vi "generateBarPosAreaQuad.vi"(7 "Number of Defenders\nWithout Duelist":i32, 8 "error in (no error)":errorcluster, 10 "Game":refnum<class "Game.lvclass">, 11 "Utilities in":refnum<class "Utilities.lvclass">) -> (0 "error out":errorcluster, 1 "Pos Centers Back":dbl[][](array[numeric]), 2 "Game out":refnum<class "Game.lvclass">, 3 "Utilities out":refnum<class "Utilities.lvclass">)   [LabVIEW 2020, in "Utilities.lvclass"]
uses:
  Utilities.lvclass
  Game_class/Game.lvclass
  Game_class/Game.lvclass/Game.ctl
  Events_class/Events.lvclass/Events.ctl
  Object_class/Object.lvclass/Object.ctl
  Game_class/Read EventsRef.vi
  Game_class/Read FieldRef.vi
  Game_class/Read BallRef.vi
  Object_class/Read x.vi
  Object_class/Read y.vi
  Events_class/Read ball_out.vi
  Events_class/Read ball_out_of_vision.vi
  Ball_class/Ball.lvclass
  Events_class/Events.lvclass
  Field_class/Field.lvclass
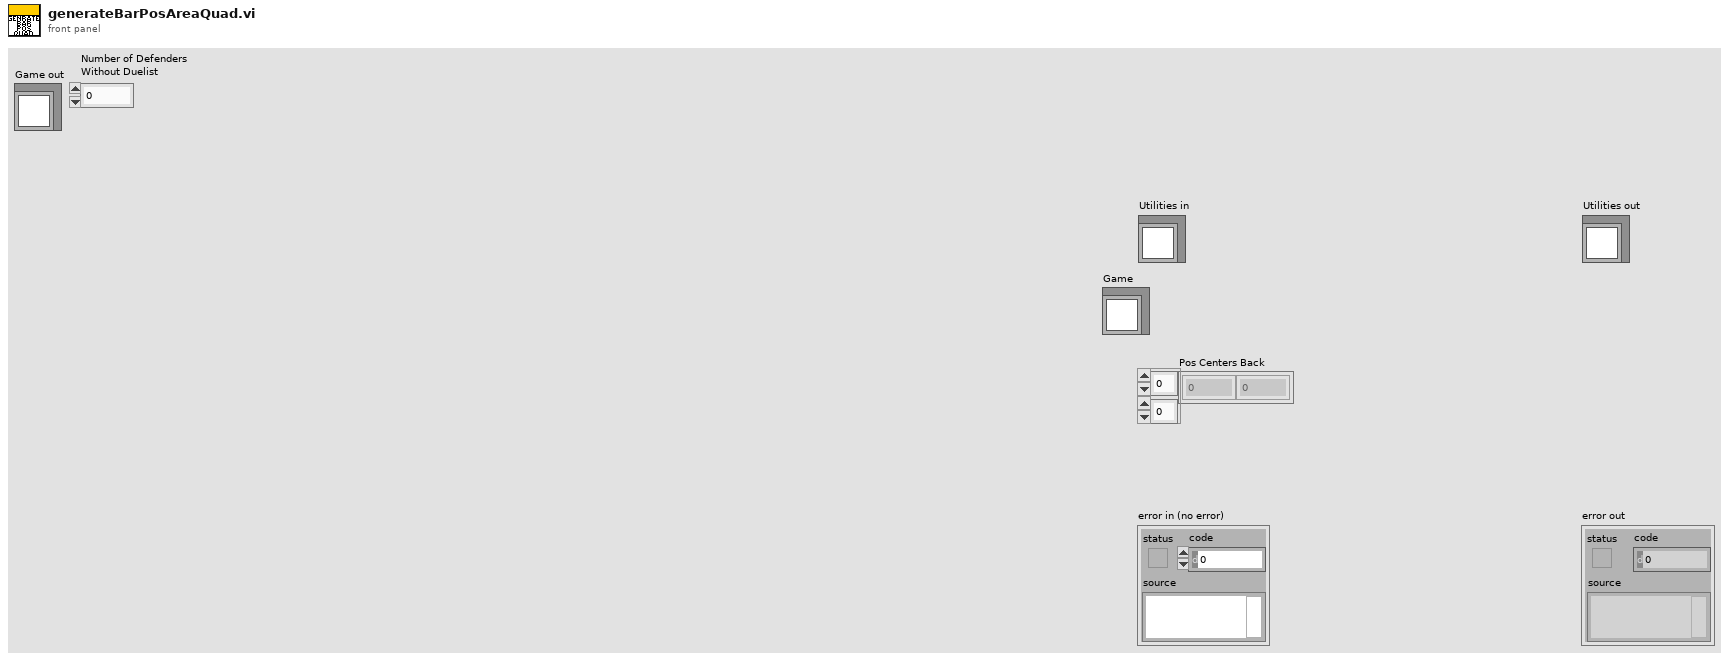
[diagram p1: front panel]
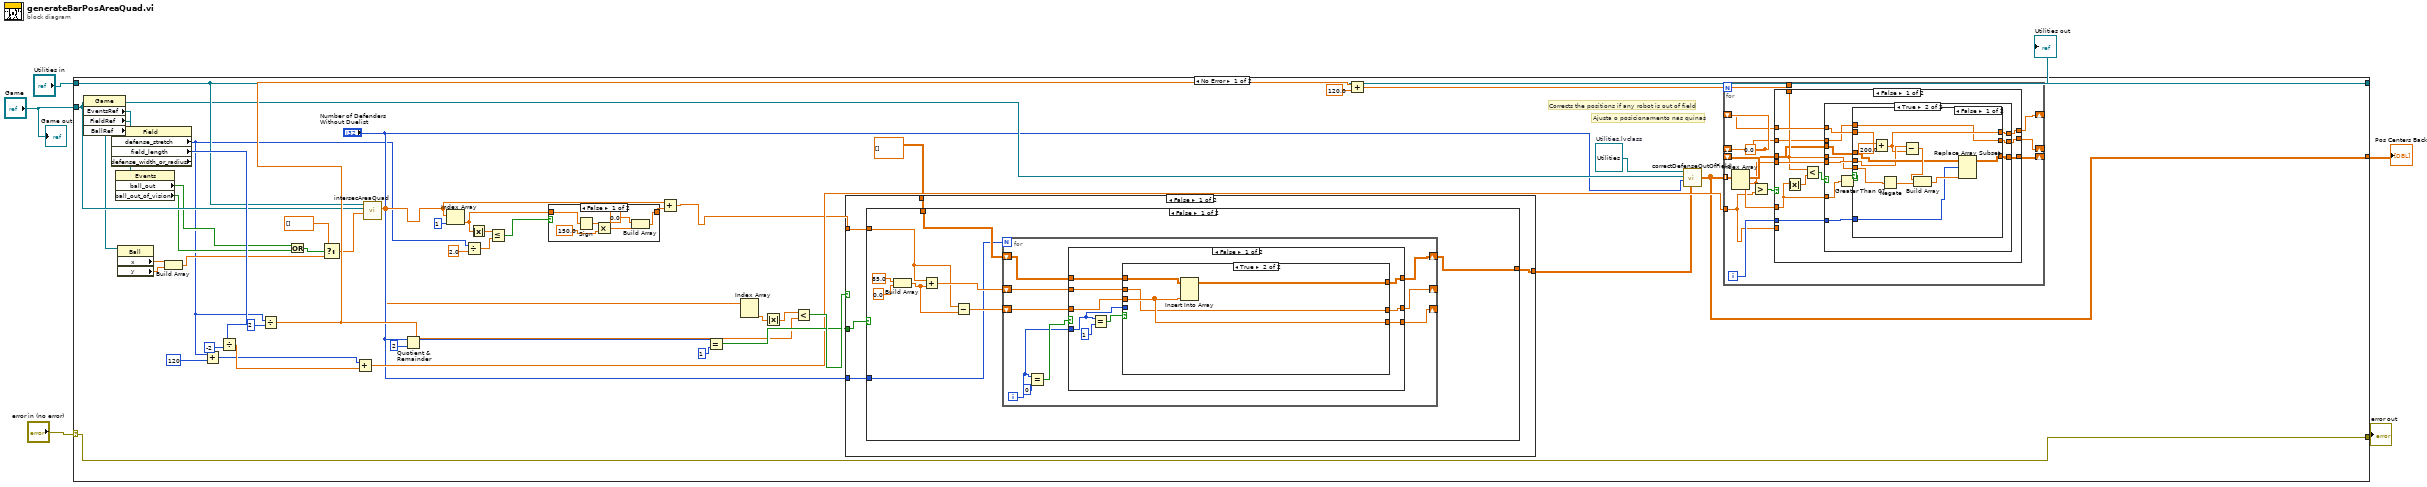
[diagram p0: block diagram]
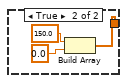
[diagram p2: hidden frame]
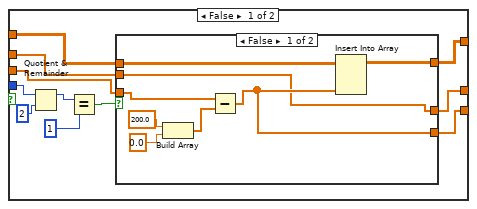
[diagram p3: hidden frame]
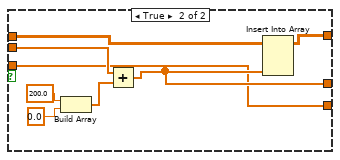
[diagram p4: hidden frame]
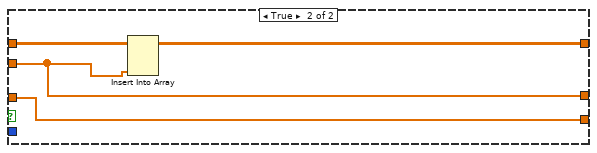
[diagram p5: hidden frame]
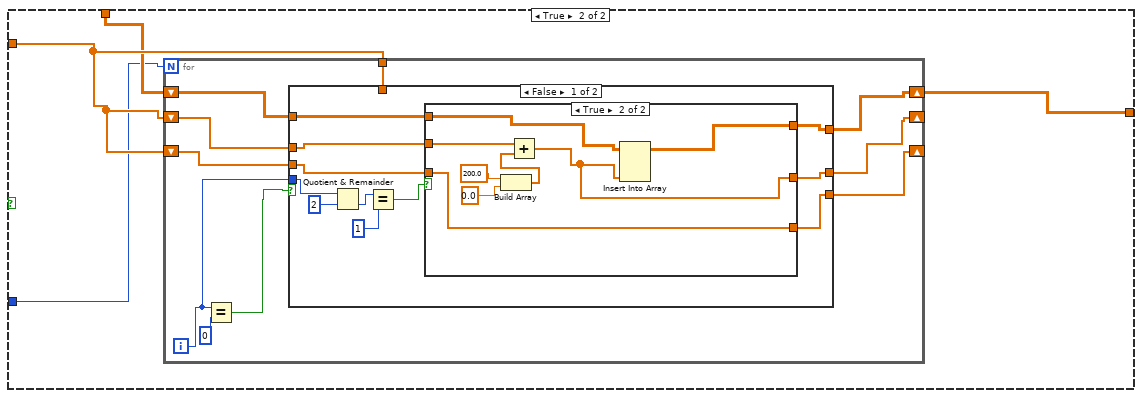
[diagram p6: hidden frame]
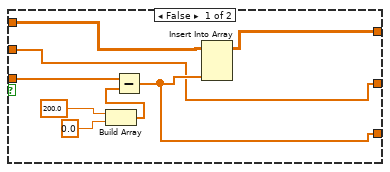
[diagram p7: hidden frame]
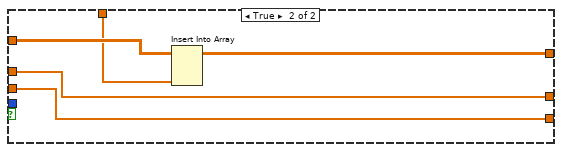
[diagram p8: hidden frame]
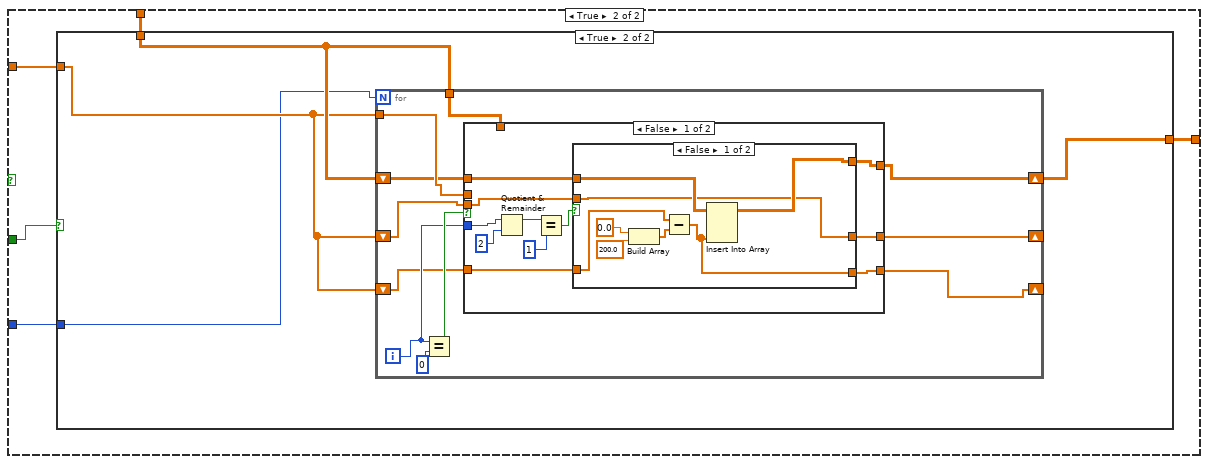
[diagram p9: hidden frame]
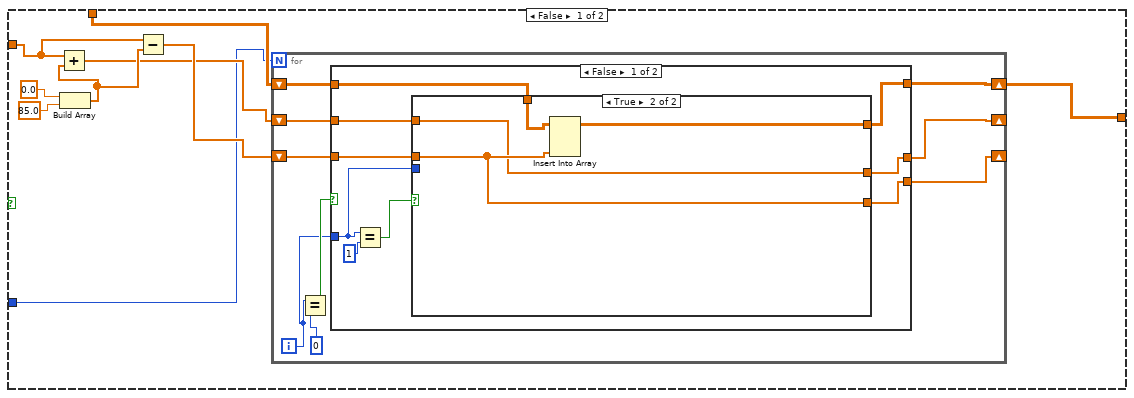
[diagram p10: hidden frame]
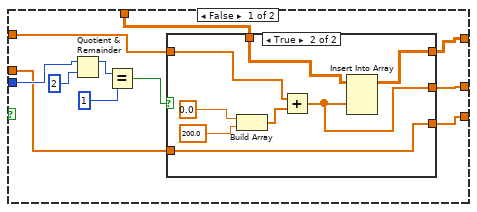
[diagram p11: hidden frame]
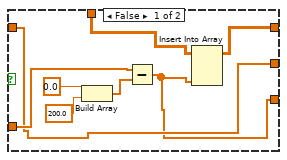
[diagram p12: hidden frame]
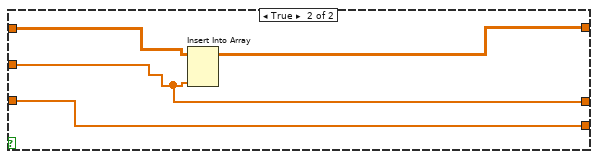
[diagram p13: hidden frame]
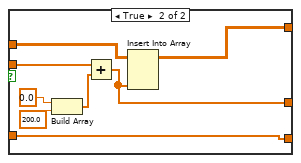
[diagram p14: hidden frame]
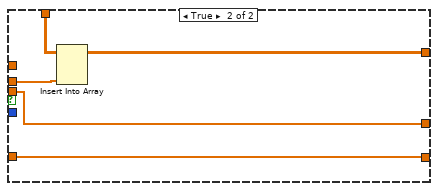
[diagram p15: hidden frame]
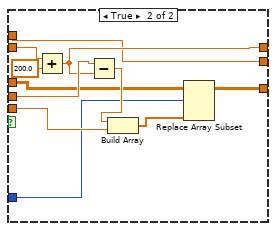
[diagram p17: hidden frame]
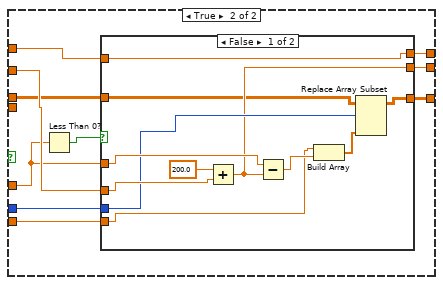
[diagram p18: hidden frame]
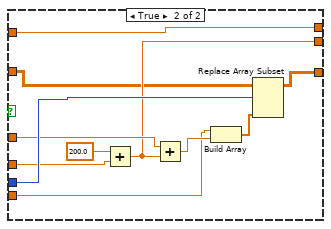
[diagram p19: hidden frame]
diagram:
  n1 = case shown="No Error" "error in (no error)" {
    selector: "error in (no error)" -> [w53 w385]
    tunnel: [w53 w385] -> w5
    tunnel: "Utilities in" -> [w33 w384]
    tunnel: [w33 w384] -> w3
    tunnel: "Game" -> [w29 _]
    tunnel: [w7 _] -> w2
    frame No Error {
      w30 = refnum<class "Utilities.lvclass"> refnum  # Utilities.lvclass
      w43 = 0.0
      # "Ajusta o posicionamento nas quinas"
      # "Corrects the positions if any robot is out of field"
      n2 = property class="Game"(reference=w29) -> ("EventsRef"=w25:refnum<class "Events.lvclass">, "FieldRef"=w35:refnum<class "Field.lvclass">, "BallRef"=w28:refnum<class "Ball.lvclass">)  [unwired: 1 in, 2 out]
      n3 = property class="Field" props=["defense_stretch", "field_length", "defense_width_or_radius"](reference=w35) -> ("defense_stretch"=w8:i32, "field_length"=w34:i32)  [unwired: 1 in, 3 out]
      n4 = property class="Events"(reference=w25) -> ("ball_out"=w24:bool, "ball_out_of_vision"=w23:bool)  [unwired: 1 in, 2 out]
      n5 = property class="Ball"(reference=w28) -> ("x"=w27:dbl, "y"=w26:dbl)  [unwired: 1 in, 2 out]
      n6 = Build Array(w27, w26) -> (w21:dbl[])
      n7 = Add(x=w8, y=u32 120) -> (x+y=w37:u32)
      n8 = Divide(x=w34, y=-2) -> (x/y=w40:dbl)
      n9 = Divide(x=w8, y=u32 2) -> (x/y=w38:dbl)
      n10 = Or(x=w24, y=w23) -> (x .or. y?=w22:bool)
      n11 = Select(t=dbl[] [], s=w22, f=w21) -> (s? t:f=w20:dbl[])
      n12 = Add(x=w37, y=w40) -> (x+y=w41:dbl)
      n13 = call "intersecAreaQuad.vi"("Ball/Enemy\nPosition"=w20, "Game"=w29, "Utilities in"=w33) -> ("Pos de Interseção"=w10:dbl[])  [unwired: 6 in, 2 out]
      n14 = Quotient & Remainder(x="Number of Defenders\nWithout Duelist", y=2) -> (x-y*floor(x/y)=w47:i32)  [unwired: 1 out]
      n15 = Index Array(array=w10, index=1) -> (element=w11:dbl)
      n16 = Divide(x=w8, y=2.0) -> (x/y=w14:dbl)
      n17 = Absolute Value(x=w11) -> (abs(x)=w15:dbl)
      n18 = Less Or Equal?(x=w15, y=w14) -> (x <= y?=w12:bool)
      n19 = case shown="False" w12 {
        tunnel: [w58 w62] -> w17
        tunnel: w11 -> [w54 _]
        frame False {
          n20 = Sign(1:w54) -> (0:w57:dbl)
          n21 = Multiply(x=w57, y=150.0) -> (x*y=w55:dbl)
          n22 = Build Array(0.0, w55) -> (w58:dbl[])
        }
        frame True {
          n23 = Build Array(150.0, 0.0) -> (w62:dbl[])
        }
      }
      n24 = Add(x=w10, y=w17) -> (x+y=w9:dbl[])
      n25 = Equal?(x=w47, y=1) -> (x = y?=w45:bool)
      n26 = Index Array(array=w10) -> (element #2=w51:dbl)  [unwired: 2 in, 1 out]
      n27 = Absolute Value(x=w51) -> (abs(x)=w50:dbl)
      n28 = Less?(x=w50, y=w38) -> (x < y?=w49:bool)
      n29 = case shown="False" w49 {
        tunnel: w45 -> [w67 w180]
        tunnel: w9 -> [w66 w179]
        tunnel: dbl[][] [] -> [w64 w178]
        tunnel: [w65 w177] -> w31
        tunnel: "Number of Defenders\nWithout Duelist" -> [w63 w176]
        frame False {
          n30 = case shown="False" w67 {
            tunnel: w64 -> [w70 w131]
            tunnel: w66 -> [w73 w133]
            tunnel: [w69 w132] -> w65
            tunnel: w63 -> [w68 w130]
            frame False {
              n31 = Build Array(85.0, 0.0) -> (w72:dbl[])
              n32 = Add(x=w73, y=w72) -> (x+y=w74:dbl[])
              n33 = Subtract(x=w73, y=w72) -> (x-y=w71:dbl[])
              n34 = for {
                N: w68 -> [_]
                shift-right: [w80] -> _
                shift-left: w74 -> [w82]
                shift-right: [w79] -> _
                shift-left: w71 -> [w78]
                shift-right: [w81] -> w69
                shift-left: w70 -> [w83]
                i -> [w77]
                n35 = Equal?(x=w77, y=0) -> (x = y?=w84:bool)
                n36 = case shown="False" w84 {
                  tunnel: w83 -> [w92 w129]
                  tunnel: w82 -> [w88 w127]
                  tunnel: [w87 w128] -> w81
                  tunnel: [w89 w127] -> w80
                  tunnel: [w90 w126] -> w79
                  tunnel: w78 -> [w91 w126]
                  tunnel: w77 -> [w86 _]
                  frame False {
                    n37 = Equal?(x=w86, y=1) -> (x = y?=w93:bool)
                    n38 = case shown="True" w93 {
                      tunnel: w92 -> [w100 w125]
                      tunnel: w91 -> [w95 w124]
                      tunnel: [w96 w124] -> w90
                      tunnel: [w97 w123] -> w89
                      tunnel: w88 -> [w99 w123]
                      tunnel: [w98 w122] -> w87
                      tunnel: w86 -> [w105 _]
                      frame False {
                        n39 = Quotient & Remainder(x=w105, y=2) -> (x-y*floor(x/y)=w103:i32)  [unwired: 1 out]
                        n40 = Equal?(x=w103, y=1) -> (x = y?=w101:bool)
                        n41 = case shown="False" w101 {
                          tunnel: w100 -> [w112 w121]
                          tunnel: w99 -> [w106 w117]
                          tunnel: [w113 w116] -> w98
                          tunnel: [w106 w115] -> w97
                          tunnel: [w107 w114] -> w96
                          tunnel: w95 -> [w108 w114]
                          frame False {
                            n42 = Build Array(200.0, 0.0) -> (w109:dbl[])
                            n43 = Subtract(x=w108, y=w109) -> (x-y=w107:dbl[])
                            n44 = Insert Into Array(array=w112, new element=w107) -> (w113:dbl[][])  [unwired: 2 in]
                          }
                          frame True {
                            n45 = Build Array(200.0, 0.0) -> (w118:dbl[])
                            n46 = Add(x=w117, y=w118) -> (x+y=w115:dbl[])
                            n47 = Insert Into Array(array=w121, new element=w115) -> (w116:dbl[][])  [unwired: 2 in]
                          }
                        }
                      }
                      frame True {
                        n48 = Insert Into Array(array=w125, new element=w124) -> (w122:dbl[][])  [unwired: 2 in]
                      }
                    }
                  }
                  frame True {
                    n49 = Insert Into Array(array=w129, new element=w127) -> (w128:dbl[][])  [unwired: 2 in]
                  }
                }
              }
            }
            frame True {
              n50 = for {
                N: w130 -> [_]
                shift-right: [w139] -> w132
                shift-left: w131 -> [w141]
                shift-right: [w137] -> _
                shift-left: w133 -> [w136]
                shift-right: [w135] -> _
                shift-left: w133 -> [w134]
                tunnel: w133 -> [w140]
                i -> [w138]
                n51 = Equal?(x=w138, y=0) -> (x = y?=w142:bool)
                n52 = case shown="False" w142 {
                  tunnel: w141 -> [w149 w175]
                  tunnel: w140 -> [_ w174]
                  tunnel: [w148 w173] -> w139
                  tunnel: w138 -> [w154 _]
                  tunnel: [w145 w172] -> w137
                  tunnel: w136 -> [w150 w172]
                  tunnel: [w146 w171] -> w135
                  tunnel: w134 -> [w147 w171]
                  frame False {
                    n53 = Quotient & Remainder(x=w154, y=2) -> (floor(x/y)=w152:i32)  [unwired: 1 out]
                    n54 = Equal?(x=w152, y=1) -> (x = y?=w144:bool)
                    n55 = case shown="True" w144 {
                      tunnel: w150 -> [w156 w168]
                      tunnel: w149 -> [w159 w166]
                      tunnel: [w158 w165] -> w148
                      tunnel: w147 -> [w160 w164]
                      tunnel: [w157 w164] -> w146
                      tunnel: [w156 w163] -> w145
                      frame False {
                        n56 = Build Array(200.0, 0.0 ("element")) -> (w161:dbl[])
                        n57 = Subtract(x=w160, y=w161) -> (x-y=w157:dbl[])
                        n58 = Insert Into Array(array=w159, new element=w157) -> (w158:dbl[][])  [unwired: 2 in]
                      }
                      frame True {
                        n59 = Build Array(200.0, 0.0) -> (w167:dbl[])
                        n60 = Add(x=w168, y=w167) -> (x+y=w163:dbl[])
                        n61 = Insert Into Array(array=w166, new element=w163) -> (w165:dbl[][])  [unwired: 2 in]
                      }
                    }
                  }
                  frame True {
                    n62 = Insert Into Array(array=w175, new element=w174) -> (w173:dbl[][])  [unwired: 2 in]
                  }
                }
              }
            }
          }
        }
        frame True {
          n63 = case shown="True" w180 {
            tunnel: w179 -> [w187 w245]
            tunnel: w178 -> [w182 w246]
            tunnel: [w183 w244] -> w177
            tunnel: w176 -> [w181 w243]
            frame False {
              n64 = Build Array(0.0, 85.0) -> (w186:dbl[])
              n65 = Add(x=w187, y=w186) -> (x+y=w184:dbl[])
              n66 = Subtract(x=w187, y=w186) -> (x-y=w185:dbl[])
              n67 = for {
                N: w181 -> [_]
                shift-right: [w190] -> _
                shift-left: w184 -> [w195]
                shift-right: [w194] -> w183
                shift-left: w182 -> [w196]
                shift-right: [w191] -> _
                shift-left: w185 -> [w192]
                i -> [w193]
                n68 = Equal?(x=w193, y=0) -> (x = y?=w197:bool)
                n69 = case shown="False" w197 {
                  tunnel: w196 -> [w205 w242]
                  tunnel: w195 -> [w200 w239]
                  tunnel: [w203 w241] -> w194
                  tunnel: w193 -> [w199 _]
                  tunnel: w192 -> [w204 w240]
                  tunnel: [w202 w240] -> w191
                  tunnel: [w201 w239] -> w190
                  frame False {
                    n70 = Equal?(x=w199, y=1) -> (x = y?=w206:bool)
                    n71 = case shown="True" w206 {
                      tunnel: w205 -> [w213 w238]
                      tunnel: w204 -> [w209 w236]
                      tunnel: [w212 w237] -> w203
                      tunnel: [w210 w236] -> w202
                      tunnel: [w211 w235] -> w201
                      tunnel: w200 -> [w214 w235]
                      tunnel: w199 -> [w218 _]
                      frame False {
                        n72 = Quotient & Remainder(x=w218, y=2) -> (x-y*floor(x/y)=w208:i32)  [unwired: 1 out]
                        n73 = Equal?(x=w208, y=1) -> (x = y?=w215:bool)
                        n74 = case shown="True" w215 {
                          tunnel: w214 -> [w220 w231]
                          tunnel: w213 -> [w221 w230]
                          tunnel: [w222 w229] -> w212
                          tunnel: [w220 w228] -> w211
                          tunnel: [w219 w227] -> w210
                          tunnel: w209 -> [w223 w227]
                          frame False {
                            n75 = Build Array(0.0, 200.0) -> (w226:dbl[])
                            n76 = Subtract(x=w223, y=w226) -> (x-y=w219:dbl[])
                            n77 = Insert Into Array(array=w221, new element=w219) -> (w222:dbl[][])  [unwired: 2 in]
                          }
                          frame True {
                            n78 = Build Array(0.0, 200.0) -> (w232:dbl[])
                            n79 = Add(x=w231, y=w232) -> (x+y=w228:dbl[])
                            n80 = Insert Into Array(array=w230, new element=w228) -> (w229:dbl[][])  [unwired: 2 in]
                          }
                        }
                      }
                      frame True {
                        n81 = Insert Into Array(array=w238, new element=w236) -> (w237:dbl[][])  [unwired: 2 in]
                      }
                    }
                  }
                  frame True {
                    n82 = Insert Into Array(array=w242, new element=w239) -> (w241:dbl[][])  [unwired: 2 in]
                  }
                }
              }
            }
            frame True {
              n83 = for {
                N: w243 -> [_]
                tunnel: w246 -> [w256]
                tunnel: w245 -> [w255]
                shift-right: [w254] -> w244
                shift-left: w246 -> [w251]
                shift-right: [w249] -> _
                shift-left: w245 -> [w250]
                shift-right: [w247] -> _
                shift-left: w245 -> [w248]
                i -> [w252]
                n84 = Equal?(x=w252, y=0) -> (x = y?=w257:bool)
                n85 = case shown="False" w257 {
                  tunnel: w256 -> [_ w289]
                  tunnel: w255 -> [_ w288]
                  tunnel: [w262 w287] -> w254
                  tunnel: w252 -> [w268 _]
                  tunnel: w251 -> [w263 _]
                  tunnel: w250 -> [w261 w286]
                  tunnel: [w260 w286] -> w249
                  tunnel: w248 -> [w259 w285]
                  tunnel: [w258 w285] -> w247
                  frame False {
                    n86 = Quotient & Remainder(x=w268, y=2) -> (x-y*floor(x/y)=w266:i32)  [unwired: 1 out]
                    n87 = Equal?(x=w266, y=1) -> (x = y?=w264:bool)
                    n88 = case shown="False" w264 {
                      tunnel: w263 -> [w272 w281]
                      tunnel: [w271 w280] -> w262
                      tunnel: w261 -> [w269 w279]
                      tunnel: [w269 w278] -> w260
                      tunnel: w259 -> [w273 w277]
                      tunnel: [w270 w277] -> w258
                      frame False {
                        n89 = Build Array(0.0, 200.0) -> (w274:dbl[])
                        n90 = Subtract(x=w273, y=w274) -> (x-y=w270:dbl[])
                        n91 = Insert Into Array(array=w272, new element=w270) -> (w271:dbl[][])  [unwired: 2 in]
                      }
                      frame True {
                        n92 = Build Array(0.0, 200.0) -> (w282:dbl[])
                        n93 = Add(x=w279, y=w282) -> (x+y=w278:dbl[])
                        n94 = Insert Into Array(array=w281, new element=w278) -> (w280:dbl[][])  [unwired: 2 in]
                      }
                    }
                  }
                  frame True {
                    n95 = Insert Into Array(array=w289, new element=w288) -> (w287:dbl[][])  [unwired: 2 in]
                  }
                }
              }
            }
          }
        }
      }
      n96 = Add(x=w38, y=120.0) -> (x+y=w36:dbl)
      n97 = call "correctDefenseOutOfField.vi"("Pos Centers Back in"=w31, "Number of Defenders\nWithout Duelist"="Number of Defenders\nWithout Duelist", "Game"=w29, "Utilities in"=w30) -> ("Pos Centers Back out"=w7:dbl[][])  [unwired: 5 in, 2 out]
      n98 = for {
        tunnel: w7 -> [w300] mode=indexing
        tunnel: w41 -> [w297]
        shift-right: [w296] -> _
        shift-left: w43 -> [w298]
        shift-right: [w294] -> _
        shift-left: w7 -> [w295]
        tunnel: w36 -> [w293]
        shift-right: [w290] -> _
        shift-left: w43 -> [w292]
        i -> [w299]
        n99 = Index Array(array=w300) -> (element #1=w291:dbl, element #2=w301:dbl)  [unwired: 2 in]
        n100 = Greater?(x=w291, y=w297) -> (0:w302:bool)
        n101 = case shown="False" w302 {
          tunnel: w301 -> [w312 w358]
          tunnel: w299 -> [w307 w360]
          tunnel: w298 -> [w304 w359]
          tunnel: w297 -> [_ w357]
          tunnel: [w303 w356] -> w296
          tunnel: w295 -> [w306 w355]
          tunnel: [w305 w354] -> w294
          tunnel: w293 -> [w308 _]
          tunnel: w292 -> [w311 w352]
          tunnel: w291 -> [w310 _]
          tunnel: [w309 w353] -> w290
          frame False {
            n102 = Absolute Value(x=w312) -> (abs(x)=w314:dbl)
            n103 = Less?(x=w308, y=w314) -> (x < y?=w313:bool)
            n104 = case shown="True" w313 {
              tunnel: w312 -> [_ w328]
              tunnel: w311 -> [w316 w326]
              tunnel: w310 -> [_ w325]
              tunnel: [w316 w324] -> w309
              tunnel: w308 -> [_ w323]
              tunnel: w307 -> [_ w322]
              tunnel: w306 -> [w317 w321]
              tunnel: [w317 w320] -> w305
              tunnel: w304 -> [w315 w319]
              tunnel: [w315 w318] -> w303
              frame False {
              }
              frame True {
                n105 = Greater Than 0?(x=w328) -> (x > 0?=w327:bool)
                n106 = case shown="False" w327 {
                  tunnel: w326 -> [w335 w351]
                  tunnel: w325 -> [w334 w349]
                  tunnel: [w331 w348] -> w324
                  tunnel: w323 -> [w332 w346]
                  tunnel: w322 -> [w329 w345]
                  tunnel: w321 -> [w336 w343]
                  tunnel: [w337 w342] -> w320
                  tunnel: w319 -> [w330 w341]
                  tunnel: [w330 w341] -> w318
                  frame False {
                    n107 = Add(x=w335, y=200.0) -> (x+y=w331:dbl)
                    n108 = Negate(x=w332) -> (-x=w333:dbl)
                    n109 = Subtract(x=w334, y=w331) -> (x-y=w339:dbl)
                    n110 = Build Array(w339, w333) -> (w338:dbl[])
                    n111 = Replace Array Subset(array=w336, new element=w338, index (row)=w329) -> (w337:dbl[][])  [unwired: 1 in]
                  }
                  frame True {
                    n112 = Add(x=w351, y=200.0) -> (x+y=w348:dbl)
                    n113 = Subtract(x=w349, y=w348) -> (x-y=w347:dbl)
                    n114 = Build Array(w347, w346) -> (w344:dbl[])
                    n115 = Replace Array Subset(array=w343, new element=w344, index (row)=w345) -> (w342:dbl[][])  [unwired: 1 in]
                  }
                }
              }
            }
          }
          frame True {
            n116 = Less Than 0?(x=w358) -> (x < 0?=w361:bool)
            n117 = case shown="False" w361 {
              tunnel: w360 -> [w368 w383]
              tunnel: w359 -> [w370 w382]
              tunnel: w358 -> [w369 w380]
              tunnel: w357 -> [w367 w377]
              tunnel: [w366 w376] -> w356
              tunnel: w355 -> [w365 w375]
              tunnel: [w364 w374] -> w354
              tunnel: [w363 w373] -> w353
              tunnel: w352 -> [w363 w373]
              frame False {
                n118 = Add(x=200.0, y=w370) -> (x+y=w366:dbl)
                n119 = Subtract(x=w369, y=w366) -> (x-y=w372:dbl)
                n120 = Build Array(w367, w372) -> (w371:dbl[])
                n121 = Replace Array Subset(array=w365, new element=w371, index (row)=w368) -> (w364:dbl[][])  [unwired: 1 in]
              }
              frame True {
                n122 = Add(x=200.0, y=w382) -> (x+y=w376:dbl)
                n123 = Add(x=w380, y=w376) -> (x+y=w379:dbl)
                n124 = Build Array(w377, w379) -> (w378:dbl[])
                n125 = Replace Array Subset(array=w375, new element=w378, index (row)=w383) -> (w374:dbl[][])  [unwired: 1 in]
              }
            }
          }
        }
      }
    }
    frame Error {
    }
  }
  "error out" <- w5
  "Utilities out" <- w3
  "Pos Centers Back" <- w2
  "Game out" <- "Game"
